vi "4461 - Lockin Engine.vi"(4 "order":i32=2, 6 "TC (s)":dbl=0.5, 9 "sampling info":cluster{"Fs":dbl, "#s":dbl}, 10 "Reference In":waveform(dbl)[](array[waveform]), 11 "Signal in":waveform(dbl)[](array[waveform])) -> (0 "filter fC (Hz)":dbl=0.3183098861837907, 3 "Results (X,Y,R,Theta)":dbl[][](array[numeric]))   [LabVIEW 2016, in "LockinDSP.lvclass"]
uses:
  LockinDSP.lvclass
  <vilib>/Analysis/baseanly.llb/Mean (DBL).vi
  <vilib>/Analysis/NI_AALBase.lvlib
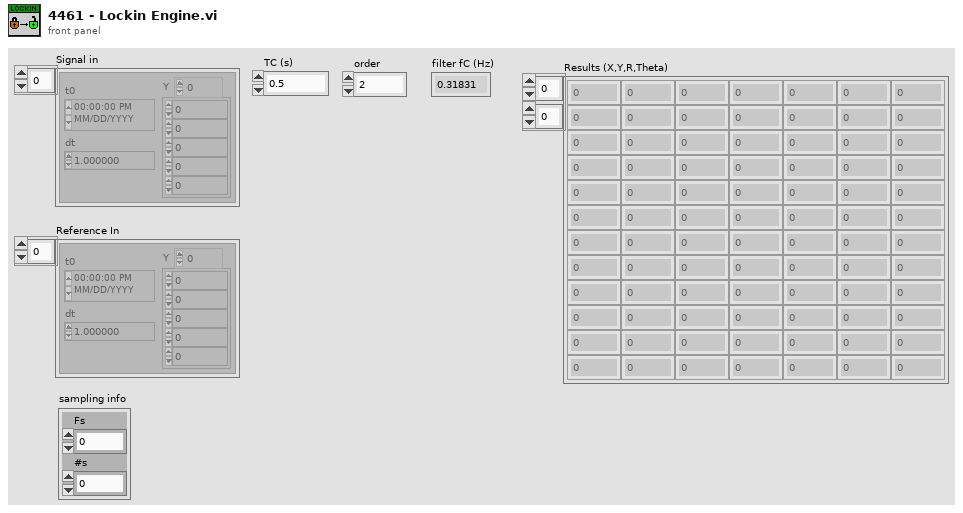
[diagram p1: front panel]
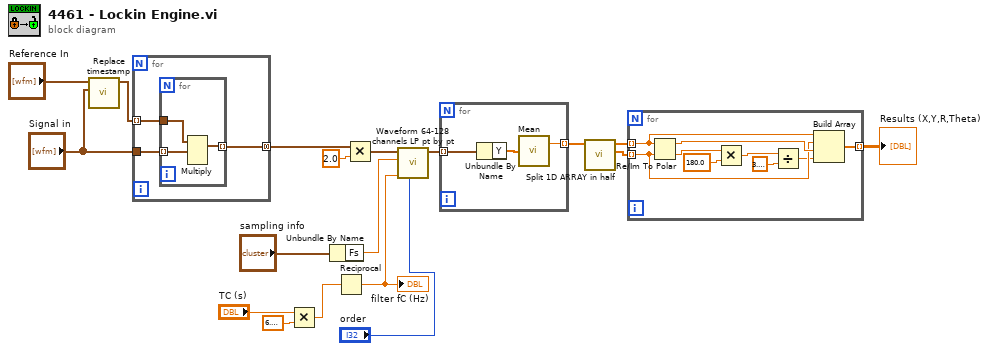
[diagram p0: block diagram]
diagram:
  n1 = call "Replace timestamp.vi"("Array in"="Signal in", "Array 2"="Reference In") -> ("Array"=w8:waveform(dbl)[])  [unwired: 9 in]
  n2 = for {
    tunnel: [w21] -> w1 mode=concatenating
    tunnel: w8 -> [w20] mode=indexing
    tunnel: "Signal in" -> [w19]
    n3 = for {
      tunnel: w19 -> [w23] mode=indexing
      tunnel: w20 -> [w22]
      tunnel: [w24] -> w21 mode=indexing
      n4 = Multiply(1:w23, 2:w22) -> (0:w24:waveform(dbl))  [unwired: 1 in, 1 out]
    }
  }
  n5 = Multiply(x="TC (s)", y=6.283185307179586) -> (x*y=w5:dbl)
  n6 = Unbundle By Name("sampling info") -> ("Fs"=w16:dbl)
  n7 = Reciprocal(x=w5) -> (1/x=w10:dbl)
  "filter fC (Hz)" <- w10
  n8 = Multiply(x=w1, y=2.0) -> (x*y=w18:waveform(dbl)[])
  n9 = call "Waveform 64-128 channels LP pt by pt.vi"("order"="order", "fl"=w10, "fs"=w16, "Array in"=w18) -> ("Array out"=w11:waveform(dbl)[])  [unwired: 7 in]
  n10 = for {
    tunnel: [w26] -> w12 mode=indexing
    tunnel: w11 -> [w25] mode=indexing
    n11 = Unbundle By Name(w25) -> ("Y"=w27:dbl[])
    n12 = call-poly <vilib>:"Mean.vi"("X"=w27) -> ("mean"=w26:dbl)  [unwired: 1 out]
  }
  n13 = call "Split 1D ARRAY in half.vi"("Array in"=w12) -> ("Array out"=w3:dbl[], "Array 3"=w2:dbl[])  [unwired: 9 in]
  n14 = for {
    tunnel: w2 -> [w33] mode=indexing
    tunnel: w3 -> [w35] mode=indexing
    tunnel: [w34] -> w7 mode=indexing
    n15 = Re/Im To Polar(2:w35, 3:w33) -> (0:w31:dbl, 1:w36:dbl)
    n16 = Multiply(x=w31, y=180.0) -> (x*y=w32:dbl)
    n17 = Divide(x=w32, y=3.141592653589793) -> (x/y=w28:dbl)
    n18 = Build Array(w33, w35, w36, w28) -> (w34:dbl[])
  }
  "Results (X,Y,R,Theta)" <- w7
